vi "Set Title.vi"(10 "Title":string, 11 "Bark in":refnum<class "Bark.lvclass">) -> (3 "Bark out":refnum<class "Bark.lvclass">)   [LabVIEW 2016, in "Bark.lvlib" / "Bark.lvclass"]
uses:
  Bark.lvclass
  Bark.lvclass/Bark.ctl
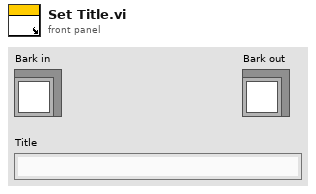
[diagram p1: front panel]
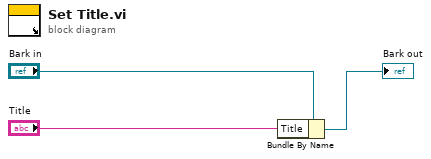
[diagram p0: block diagram]
diagram:
  n1 = Bundle By Name(cluster="Bark in", "Title"="Title") -> (→"Bark out":refnum<class "Bark.lvclass">)
